vi "RANGE Meter Bank Select 2.vi"(8 "Error In":errorcluster, 10 "Meter Data":T2={"Meter 1"={"Meter Size"=0.0, "DAQ Output (Voltage)"=0.0, "Reference (Voltage)"=0.0, "Meter Present"=FALSE, "Meter Visa"="COM3", "Gas Type"="12", "SLPM Error @ Zero"=0.0, "Gas Mix Number"="", "Set STP Register"=FALSE, "Measurement Units"={"Software Rev"="", "Model Number"="", "Manufacturer Info"="", "Software Sub-Rev"="", "Board Rev"="", "Units of Measure Input"={"Abs. Pressure"="", "Gauge/Diff. Press."="", "Barometric Press."="", "Temperature"="", "Volume"="", "Mass"="", "Setpoint"="", "Valve Drive"="", "Totalizer"="", "Tot. Timer"="", "Tot. Avg. Flow"="", "Tot. Peak Flow"=""}}, "Data Frame Format"={"Absolute Pressure"=FALSE, "Gauge/Diff. Pressure"=FALSE, "Barometric Pressure"=FALSE, "Temperature"=FALSE, "Volumetric"=FALSE, "Mass"=FALSE, "Setpoint"=FALSE, "Valve Drive"=FALSE, "Totalizer"=FALSE, "Totalizer Timer"=FALSE, "Totalizer Average Flow"=FALSE, "Totalizer Peak Flow"=FALSE, "Gas Selected"=FALSE, "Tot. Timer Format"=0}}, "Meter 2"={"Meter Size"=0.0, "DAQ Output (Voltage)"=0.0, "Reference (Voltage)"=0.0, "Meter Present"=FALSE, "Meter Visa"="COM3", "Gas Type"="12", "SLPM Error @ Zero"=0.0, "Gas Mix Number"="", "Set STP Register"=FALSE, "Measurement Units"={"Software Rev"="", "Model Number"="", "Manufacturer Info"="", "Software Sub-Rev"="", "Board Rev"="", "Units of Measure Input"={"Abs. Pressure"="", "Gauge/Diff. Press."="", "Barometric Press."="", "Temperature"="", "Volume"="", "Mass"="", "Setpoint"="", "Valve Drive"="", "Totalizer"="", "Tot. Timer"="", "Tot. Avg. Flow"="", "Tot. Peak Flow"=""}}, "Data Frame Format"={"Absolute Pressure"=FALSE, "Gauge/Diff. Pressure"=FALSE, "Barometric Pressure"=FALSE, "Temperature"=FALSE, "Volumetric"=FALSE, "Mass"=FALSE, "Setpoint"=FALSE, "Valve Drive"=FALSE, "Totalizer"=FALSE, "Totalizer Timer"=FALSE, "Totalizer Average Flow"=FALSE, "Totalizer Peak Flow"=FALSE, "Gas Selected"=FALSE, "Tot. Timer Format"=0}}, "Meter 3"={"Meter Size"=0.0, "DAQ Output (Voltage)"=0.0, "Reference (Voltage)"=0.0, "Meter Present"=FALSE, "Meter Visa"="COM3", "Gas Type"="12", "SLPM Error @ Zero"=0.0, "Gas Mix Number"="", "Set STP Register"=FALSE, "Measurement Units"={"Software Rev"="", "Model Number"="", "Manufacturer Info"="", "Software Sub-Rev"="", "Board Rev"="", "Units of Measure Input"={"Abs. Pressure"="", "Gauge/Diff. Press."="", "Barometric Press."="", "Temperature"="", "Volume"="", "Mass"="", "Setpoint"="", "Valve Drive"="", "Totalizer"="", "Tot. Timer"="", "Tot. Avg. Flow"="", "Tot. Peak Flow"=""}}, "Data Frame Format"={"Absolute Pressure"=FALSE, "Gauge/Diff. Pressure"=FALSE, "Barometric Pressure"=FALSE, "Temperature"=FALSE, "Volumetric"=FALSE, "Mass"=FALSE, "Setpoint"=FALSE, "Valve Drive"=FALSE, "Totalizer"=FALSE, "Totalizer Timer"=FALSE, "Totalizer Average Flow"=FALSE, "Totalizer Peak Flow"=FALSE, "Gas Selected"=FALSE, "Tot. Timer Format"=0}}, "Meter 4"={"Meter Size"=0.0, "DAQ Output (Voltage)"=0.0, "Reference (Voltage)"=0.0, "Meter Present"=FALSE, "Meter Visa"="COM3", "Gas Type"="12", "SLPM Error @ Zero"=0.0, "Gas Mix Number"="", "Set STP Register"=FALSE, "Measurement Units"={"Software Rev"="", "Model Number"="", "Manufacturer Info"="", "Software Sub-Rev"="", "Board Rev"="", "Units of Measure Input"={"Abs. Pressure"="", "Gauge/Diff. Press."="", "Barometric Press."="", "Temperature"="", "Volume"="", "Mass"="", "Setpoint"="", "Valve Drive"="", "Totalizer"="", "Tot. Timer"="", "Tot. Avg. Flow"="", "Tot. Peak Flow"=""}}, "Data Frame Format"={"Absolute Pressure"=FALSE, "Gauge/Diff. Pressure"=FALSE, "Barometric Pressure"=FALSE, "Temperature"=FALSE, "Volumetric"=FALSE, "Mass"=FALSE, "Setpoint"=FALSE, "Valve Drive"=FALSE, "Totalizer"=FALSE, "Totalizer Timer"=FALSE, "Totalizer Average Flow"=FALSE, "Totalizer Peak Flow"=FALSE, "Gas Selected"=FALSE, "Tot. Timer Format"=0}}, "Meter 5"={"Meter Size"=0.0, "DAQ Output (Voltage)"=0.0, "Reference (Voltage)"=0.0, "Meter Present"=FALSE, "Meter Visa"="COM3", "Gas Type"="12", "SLPM Error @ Zero"=0.0, "Gas Mix Number"="", "Set STP Register"=FALSE, "Measurement Units"={"Software Rev"="", "Model Number"="", "Manufacturer Info"="", "Software Sub-Rev"="", "Board Rev"="", "Units of Measure Input"={"Abs. Pressure"="", "Gauge/Diff. Press."="", "Barometric Press."="", "Temperature"="", "Volume"="", "Mass"="", "Setpoint"="", "Valve Drive"="", "Totalizer"="", "Tot. Timer"="", "Tot. Avg. Flow"="", "Tot. Peak Flow"=""}}, "Data Frame Format"={"Absolute Pressure"=FALSE, "Gauge/Diff. Pressure"=FALSE, "Barometric Pressure"=FALSE, "Temperature"=FALSE, "Volumetric"=FALSE, "Mass"=FALSE, "Setpoint"=FALSE, "Valve Drive"=FALSE, "Totalizer"=FALSE, "Totalizer Timer"=FALSE, "Totalizer Average Flow"=FALSE, "Totalizer Peak Flow"=FALSE, "Gas Selected"=FALSE, "Tot. Timer Format"=0}}, "Meter 6"={"Meter Size"=0.0, "DAQ Output (Voltage)"=0.0, "Reference (Voltage)"=0.0, "Meter Present"=FALSE, "Meter Visa"="COM3", "Gas Type"="12", "SLPM Error @ Zero"=0.0, "Gas Mix Number"="", "Set STP Register"=FALSE, "Measurement Units"={"Software Rev"="", "Model Number"="", "Manufacturer Info"="", "Software Sub-Rev"="", "Board Rev"="", "Units of Measure Input"={"Abs. Pressure"="", "Gauge/Diff. Press."="", "Barometric Press."="", "Temperature"="", "Volume"="", "Mass"="", "Setpoint"="", "Valve Drive"="", "Totalizer"="", "Tot. Timer"="", "Tot. Avg. Flow"="", "Tot. Peak Flow"=""}}, "Data Frame Format"={"Absolute Pressure"=FALSE, "Gauge/Diff. Pressure"=FALSE, "Barometric Pressure"=FALSE, "Temperature"=FALSE, "Volumetric"=FALSE, "Mass"=FALSE, "Setpoint"=FALSE, "Valve Drive"=FALSE, "Totalizer"=FALSE, "Totalizer Timer"=FALSE, "Totalizer Average Flow"=FALSE, "Totalizer Peak Flow"=FALSE, "Gas Selected"=FALSE, "Tot. Timer Format"=0}}, "Meter Bank 1"={"Flow Rate (BTU/HR)"=0.0, "ANSI Average (BTU/HR)"=0.0, "Panel Data"={"Meter Type (Gas)"="", "Heating Value (BTU/ft³)"=0.0, "Ft³ / Hr (SCFH)"=0.0, "15 Second Average (BTU/HR)"=0.0, "30 Second Average (BTU/HR)"=0.0, "Mass Flow"=0.0, "Vol. Flow"=0.0, "Gas Temperature"=0.0, "Gas Pressure"=0.0, "Tot.Flow"=0.0}, "Meter ID"="", "ANSI Rate"={"Array 1"=[], "Array 3"=[], "Array 2"=[], "Start ANSI"=FALSE, "ANSI Start Time"=0.0, "Restart ANSI"=FALSE, "15 Min ANSI Avg (BTU/hr)"=0.0, "20 Min ANSI Avg (BTU/hr)"=0.0, "25 Min ANSI Avg (BTU/hr)"=0.0, "Absolute Pressure"=0.0, "Gas Temperature"=0.0, "Volumetric Flow Rate"=0.0, "Mass Flow Rate"=0.0, "Array 4"=[], "Array 5"=[], "Gas Rate"=0.0, "15 Min Pres Avg (PSIA)"=0.0, "20 Min Pres Avg (PSIA)"=0.0, "25 Min Pres Avg (PSIA)"=0.0, "15 Min Temp Avg (°F) "=0.0, "20 Min Temp Avg (°F)"=0.0, "25 Min Temp Avg (°F)"=0.0, "15 Min Uncorrected Avg (CFH)"=0.0, "20 Min Uncorrected Avg (CFH)"=0.0, "25 Min Uncorrected Avg (CFH)"=0.0, "15 Min Corrected Avg (SCFH)"=0.0, "20 Min Corrected Avg (SCFH)"=0.0, "25 Min Corrected Avg (SCFH)"=0.0, "15 Min Complete"=FALSE, "20 Min Complete"=FALSE, "25 Min Complete"=FALSE, "Heating Value (BTU/ft³)"=0.0, "CO CO2 15 Min"=[], "CO CO2 20 Min"=[], "CO CO2 25 Min"=[], "CO CO2 Real Time"=[]}}, "Meter Bank 2"={"Flow Rate (BTU/HR)"=0.0, "ANSI Average (BTU/HR)"=0.0, "Panel Data"={"Meter Type (Gas)"="", "Heating Value (BTU/ft³)"=0.0, "Ft³ / Hr (SCFH)"=0.0, "15 Second Average (BTU/HR)"=0.0, "30 Second Average (BTU/HR)"=0.0, "Mass Flow"=0.0, "Vol. Flow"=0.0, "Gas Temperature"=0.0, "Gas Pressure"=0.0, "Tot.Flow"=0.0}, "Meter ID"="", "ANSI Rate"={"Array 1"=[], "Array 3"=[], "Array 2"=[], "Start ANSI"=FALSE, "ANSI Start Time"=0.0, "Restart ANSI"=FALSE, "15 Min ANSI Avg (BTU/hr)"=0.0, "20 Min ANSI Avg (BTU/hr)"=0.0, "25 Min ANSI Avg (BTU/hr)"=0.0, "Absolute Pressure"=0.0, "Gas Temperature"=0.0, "Volumetric Flow Rate"=0.0, "Mass Flow Rate"=0.0, "Array 4"=[], "Array 5"=[], "Gas Rate"=0.0, "15 Min Pres Avg (PSIA)"=0.0, "20 Min Pres Avg (PSIA)"=0.0, "25 Min Pres Avg (PSIA)"=0.0, "15 Min Temp Avg (°F) "=0.0, "20 Min Temp Avg (°F)"=0.0, "25 Min Temp Avg (°F)"=0.0, "15 Min Uncorrected Avg (CFH)"=0.0, "20 Min Uncorrected Avg (CFH)"=0.0, "25 Min Uncorrected Avg (CFH)"=0.0, "15 Min Corrected Avg (SCFH)"=0.0, "20 Min Corrected Avg (SCFH)"=0.0, "25 Min Corrected Avg (SCFH)"=0.0, "15 Min Complete"=FALSE, "20 Min Complete"=FALSE, "25 Min Complete"=FALSE, "Heating Value (BTU/ft³)"=0.0, "CO CO2 15 Min"=[], "CO CO2 20 Min"=[], "CO CO2 25 Min"=[], "CO CO2 Real Time"=[]}}, "Meter Bank 3"={"Flow Rate (BTU/HR)"=0.0, "ANSI Average (BTU/HR)"=0.0, "Panel Data"={"Meter Type (Gas)"="", "Heating Value (BTU/ft³)"=0.0, "Ft³ / Hr (SCFH)"=0.0, "15 Second Average (BTU/HR)"=0.0, "30 Second Average (BTU/HR)"=0.0, "Mass Flow"=0.0, "Vol. Flow"=0.0, "Gas Temperature"=0.0, "Gas Pressure"=0.0, "Tot.Flow"=0.0}, "Meter ID"="", "ANSI Rate"={"Array 1"=[], "Array 3"=[], "Array 2"=[], "Start ANSI"=FALSE, "ANSI Start Time"=0.0, "Restart ANSI"=FALSE, "15 Min ANSI Avg (BTU/hr)"=0.0, "20 Min ANSI Avg (BTU/hr)"=0.0, "25 Min ANSI Avg (BTU/hr)"=0.0, "Absolute Pressure"=0.0, "Gas Temperature"=0.0, "Volumetric Flow Rate"=0.0, "Mass Flow Rate"=0.0, "Array 4"=[], "Array 5"=[], "Gas Rate"=0.0, "15 Min Pres Avg (PSIA)"=0.0, "20 Min Pres Avg (PSIA)"=0.0, "25 Min Pres Avg (PSIA)"=0.0, "15 Min Temp Avg (°F) "=0.0, "20 Min Temp Avg (°F)"=0.0, "25 Min Temp Avg (°F)"=0.0, "15 Min Uncorrected Avg (CFH)"=0.0, "20 Min Uncorrected Avg (CFH)"=0.0, "25 Min Uncorrected Avg (CFH)"=0.0, "15 Min Corrected Avg (SCFH)"=0.0, "20 Min Corrected Avg (SCFH)"=0.0, "25 Min Corrected Avg (SCFH)"=0.0, "15 Min Complete"=FALSE, "20 Min Complete"=FALSE, "25 Min Complete"=FALSE, "Heating Value (BTU/ft³)"=0.0, "CO CO2 15 Min"=[], "CO CO2 20 Min"=[], "CO CO2 25 Min"=[], "CO CO2 Real Time"=[]}}, "Threshold Voltage (NI DAQ)"=0.0, "Use RS232 Data Collection"=FALSE, "Use Auto Switching"=FALSE}, 11 "Meter Select 2":T1 caption="Meter Select") -> (0 "Error Out":errorcluster, 2 "Unit ID":string, 3 "VISA Refnum out":refnum<visa-resource-name>)   [LabVIEW 2019]
uses:
  Type Definitions/RANGE DAQ Data Four Meters.ctl
  Type Definitions/RANGE DAQ Data.ctl
  Drivers/Omega FMA-1600A Series Gas Flow Meter/Type Definitions/FMA1600A Gas Type.ctl
  Drivers/Omega FMA-1600A Series Gas Flow Meter/Type Definitions/FMA1600A Units String.ctl
  Drivers/Alicat Gas Meter Driver/Sub-VIs/Units of Measure.ctl
  Drivers/Alicat Gas Meter Driver/Sub-VIs/Data Frame.ctl
  Type Definitions/RANGE GAS Data.ctl
  Type Definitions/RANGE Panel Data.ctl
  Type Definitions/RANGE ANSI Rate.ctl
  Type Definitions/RANGE Meter Selector 3-4.ctl
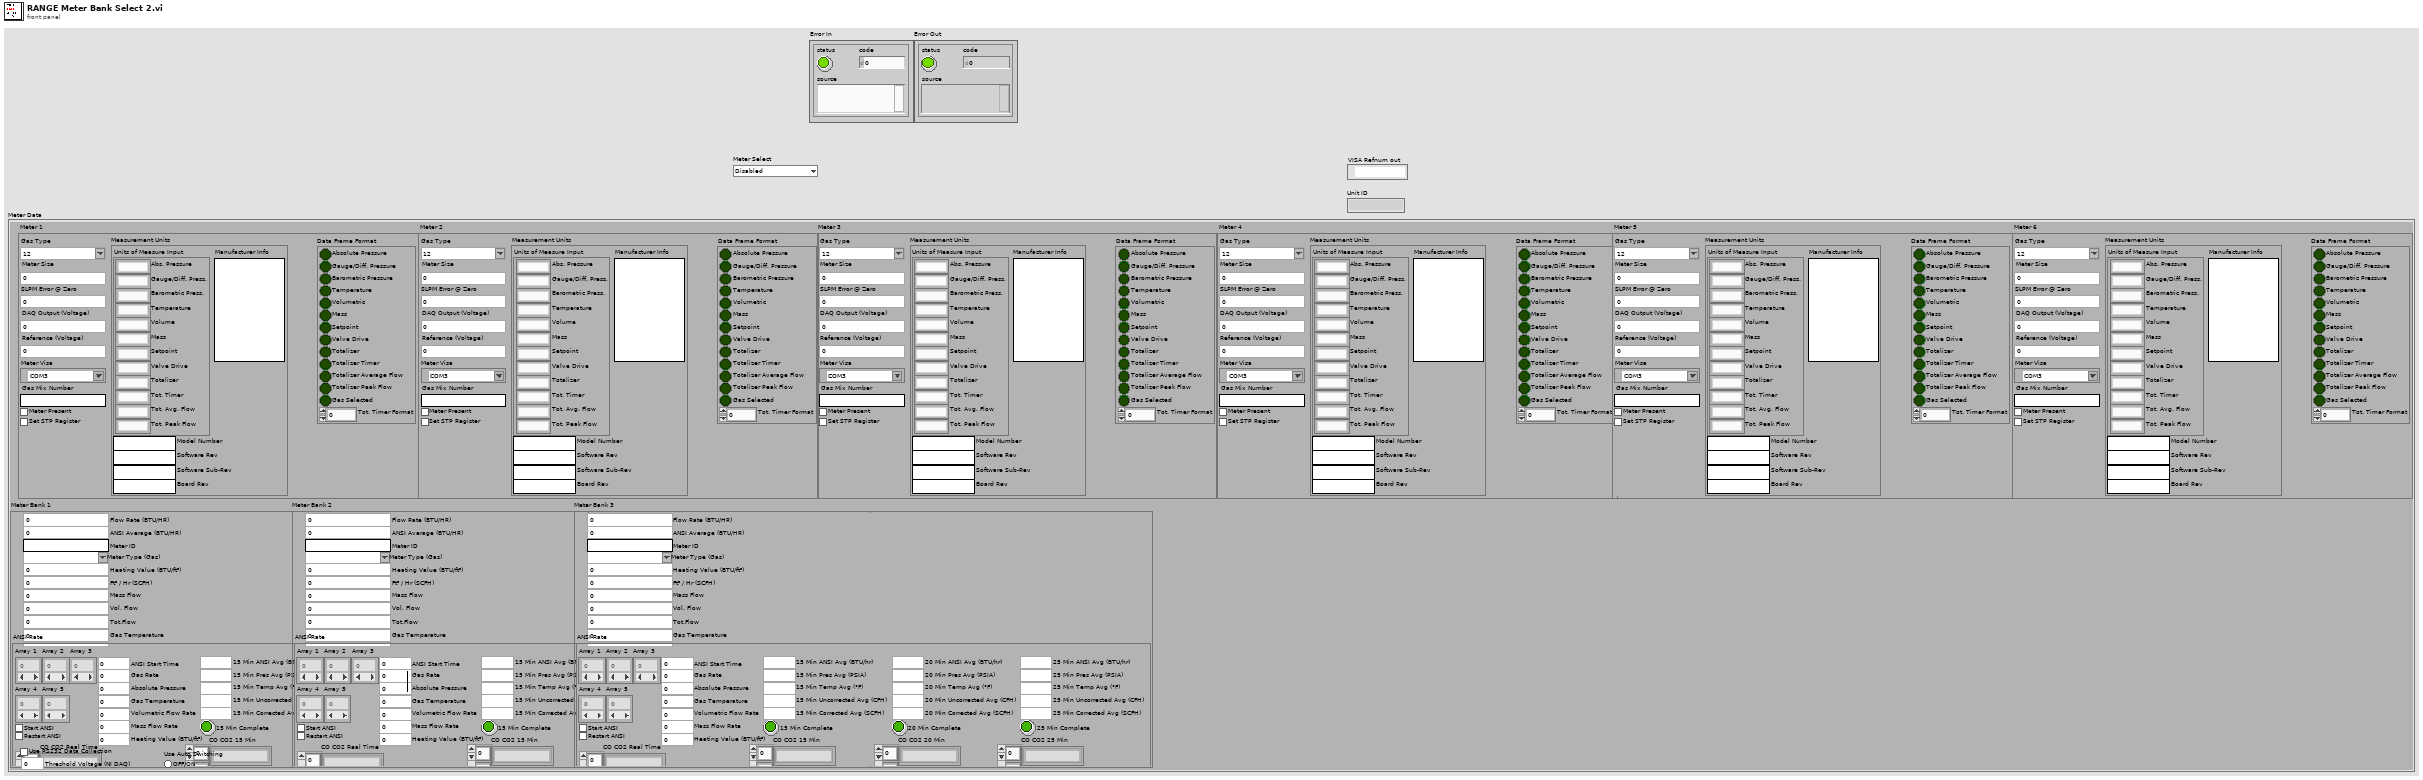
[diagram p1: front panel]
types:
  T1 = typedef "RANGE Meter Selector 3-4.ctl" = enum16{"Disabled", "Meter 3", "Meter 4", "Auto"}
  T2 = typedef "RANGE DAQ Data Four Meters.ctl" = cluster{"Meter 1":T3, "Meter 2":T3, "Meter 3":T3, "Meter 4":T3, "Meter 5":T3, "Meter 6":T3, "Meter Bank 1":T8, "Meter Bank 2":T8, "Meter Bank 3":T8, "Threshold Voltage (NI DAQ)":dbl, "Use RS232 Data Collection":bool, "Use Auto Switching":bool}
  T3 = typedef "RANGE DAQ Data.ctl" = cluster{"Meter Size":dbl, "DAQ Output (Voltage)":dbl, "Reference (Voltage)":dbl, "Meter Present":bool, "Meter Visa":refnum<visa-resource-name>, "Gas Type":T4, "SLPM Error @ Zero":dbl, "Gas Mix Number":string, "Set STP Register":bool, "Measurement Units":T5, "Data Frame Format":T7}
  T4 = typedef "FMA1600A Gas Type.ctl" = string
  T5 = typedef "FMA1600A Units String.ctl" = cluster{"Software Rev":string, "Model Number":string, "Manufacturer Info":string, "Software Sub-Rev":string, "Board Rev":string, "Units of Measure Input":T6}
  T6 = typedef "Units of Measure.ctl" = cluster{"Abs. Pressure":string, "Gauge/Diff. Press.":string, "Barometric Press.":string, "Temperature":string, "Volume":string, "Mass":string, "Setpoint":string, "Valve Drive":string, "Totalizer":string, "Tot. Timer":string, "Tot. Avg. Flow":string, "Tot. Peak Flow":string}
  T7 = typedef "Data Frame.ctl" = cluster{"Absolute Pressure":bool, "Gauge/Diff. Pressure":bool, "Barometric Pressure":bool, "Temperature":bool, "Volumetric":bool, "Mass":bool, "Setpoint":bool, "Valve Drive":bool, "Totalizer":bool, "Totalizer Timer":bool, "Totalizer Average Flow":bool, "Totalizer Peak Flow":bool, "Gas Selected":bool, "Tot. Timer Format":u16}
  T8 = typedef "RANGE GAS Data.ctl" = cluster{"Flow Rate (BTU/HR)":dbl, "ANSI Average (BTU/HR)":dbl, "Panel Data":T9, "Meter ID":string, "ANSI Rate":T10}
  T9 = typedef "RANGE Panel Data.ctl" = cluster{"Meter Type (Gas)":T4, "Heating Value (BTU/ft³)":dbl, "Ft³ / Hr (SCFH)":dbl, "15 Second Average (BTU/HR)":dbl, "30 Second Average (BTU/HR)":dbl, "Mass Flow":dbl, "Vol. Flow":dbl, "Gas Temperature":dbl, "Gas Pressure":dbl, "Tot.Flow":dbl}
  T10 = typedef "RANGE ANSI Rate.ctl" = cluster{"Array 1":dbl[], "Array 3":dbl[], "Array 2":dbl[], "Start ANSI":bool, "ANSI Start Time":dbl, "Restart ANSI":bool, "15 Min ANSI Avg (BTU/hr)":dbl, "20 Min ANSI Avg (BTU/hr)":dbl, "25 Min ANSI Avg (BTU/hr)":dbl, "Absolute Pressure":dbl, "Gas Temperature":dbl, "Volumetric Flow Rate":dbl, "Mass Flow Rate":dbl, "Array 4":dbl[], "Array 5":dbl[], "Gas Rate":dbl, "15 Min Pres Avg (PSIA)":dbl, "20 Min Pres Avg (PSIA)":dbl, "25 Min Pres Avg (PSIA)":dbl, "15 Min Temp Avg (°F) ":dbl, "20 Min Temp Avg (°F)":dbl, "25 Min Temp Avg (°F)":dbl, "15 Min Uncorrected Avg (CFH)":dbl, "20 Min Uncorrected Avg (CFH)":dbl, "25 Min Uncorrected Avg (CFH)":dbl, "15 Min Corrected Avg (SCFH)":dbl, "20 Min Corrected Avg (SCFH)":dbl, "25 Min Corrected Avg (SCFH)":dbl, "15 Min Complete":bool, "20 Min Complete":bool, "25 Min Complete":bool, "Heating Value (BTU/ft³)":dbl, "CO CO2 15 Min":string[][], "CO CO2 20 Min":string[][], "CO CO2 25 Min":string[][], "CO CO2 Real Time":string[][]}
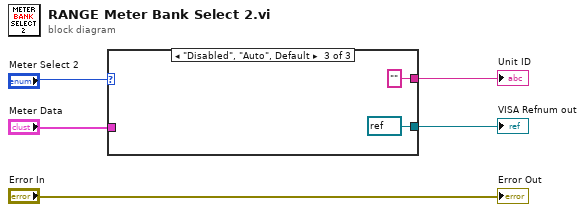
[diagram p0: block diagram]
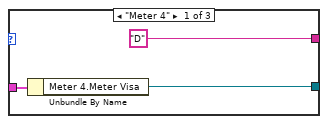
[diagram p2: hidden frame]
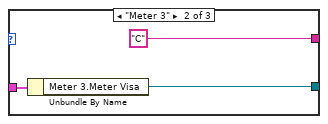
[diagram p3: hidden frame]
diagram:
  n1 = case shown="\"Disabled\", \"Auto\", Default" "Meter Select 2" {
    tunnel: ["D" "C" ""] -> w3
    tunnel: "Meter Data" -> [w7 w10 _]
    tunnel: [w6 w9 refnum<visa-resource-name> refnum ("Meter Visa")] -> w5
    frame "Meter 4" {
      n2 = Unbundle By Name(w7) -> ("Meter 4.Meter Visa"=w6:refnum<visa-resource-name>)
    }
    frame "Meter 3" {
      n3 = Unbundle By Name(w10) -> ("Meter 3.Meter Visa"=w9:refnum<visa-resource-name>)
    }
    frame "Disabled", "Auto", Default {
    }
  }
  "VISA Refnum out" <- w5
  "Unit ID" <- w3
  "Error Out" <- "Error In"
